vi "LinxPwmSetDutyCycle.vi"(8 "Error In":errorcluster, 9 "Duty Cycles":dbl[](array[numeric]), 10 "PWM Channels":u8[](array[numeric]), 11 "LINX Resource":T1) -> (0 "Error Out":errorcluster, 3 "LINX Resource":T1)   [LabVIEW 2014, in "LMH-LINX.lvlib" / "Local IO.lvlib"]
uses:
  Local IO.lvlib
  Type Defs/LINX Ref.ctl
  Type Defs/Platform.ctl
  Type Defs/Interface.ctl
  Device/Type Defs/LINX Device Config.ctl
  Device/Type Defs/TCP Config.ctl
  Device/Type Defs/Channels.ctl
  Utilties/Generate Error.vi
  <vilib>/myRIO/Instrument Drivers/Onboard IO/PWM/PWM.lvlib
  liblinxdevice.dll
  LMH-LINX.lvlib
  Device/Device.lvlib
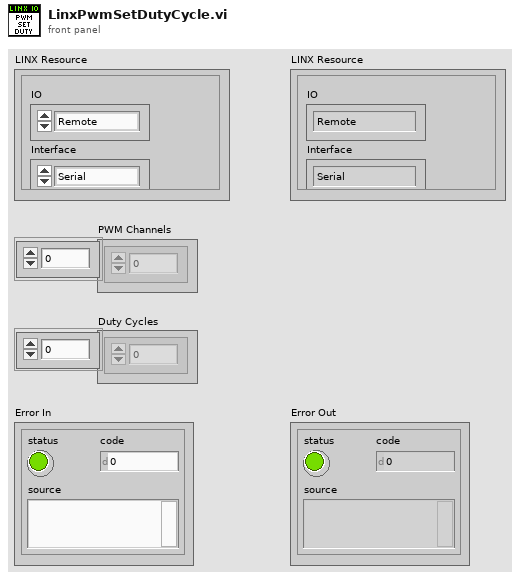
[diagram p1: front panel]
types:
  T1 = typedef "LMH-LINX.lvlib/LINX Ref.ctl" = cluster{"IO":T2, "Interface":T3, "LINX Device Config":T4}
  T2 = typedef "LMH-LINX.lvlib/Platform.ctl" = enum16{"Remote", "Local"}
  T3 = typedef "LMH-LINX.lvlib/Interface.ctl" = enum16{"Serial", "TCP"}
  T4 = typedef "LMH-LINX.lvlib/Device.lvlib/LINX Device Config.ctl" = cluster{"Interface":T3, "COM Port":refnum<visa-resource-name>, "TCP Configuration":T5, "Device Family":u8, "Device ID":u8, "Device Name":string, "TCP Ref":refnum<k5>, "Channels":T6}
  T5 = typedef "LMH-LINX.lvlib/Device.lvlib/TCP Config.ctl" = cluster{"IP Address":string, "Port":u16}
  T6 = typedef "LMH-LINX.lvlib/Channels.ctl" = cluster{"DI":u8[], "DO":u8[], "AI":u8[], "AO":u8[], "PWM":u8[], "QE":u8[], "UART":u8[], "I2C 2":u8[], "SPI":u8[], "CAN":u8[], "Servo":u8[], "AI Ref (V)":dbl, "AI Resolution (Bits)":u8, "AO Ref (V)":dbl, "AO Resolution (Bits)":u8}
  T7 = typedef "PWM.lvlib/PWM Reference.ctl" = cluster{"myRIO Reference":T8, "PWM Channels Enum":T12, "PWM Configuration":T13}
  T8 = typedef "myRIO Generic Hardware Reference.ctl" = cluster{"myRIO Model":T9, "myRIO Hardware Reference":T10}
  T9 = typedef "Hardware Version Enum.ctl" = enum16{"Unknown", "myRIO-1900", "myRIO-1950"}
  T10 = typedef "myRIO v1.0 Reference.ctl" = cluster{"Generic FPGA Reference":T11, "Allow multiple opens":bool}
  T11 = typedef "Generic FPGA Reference.ctl" = refnum<k20>
  T12 = typedef "PWM Channels Enum.ctl" = enum16{"Not Connected", "C/PWM0", "C/PWM1", "A/PWM0", "A/PWM1", "A/PWM2", "B/PWM0", "B/PWM1", "B/PWM2"}
  T13 = typedef "PWM.lvlib/PWM Configuration.ctl" = cluster{"Frequency":dbl, "Duty Cycle":dbl}
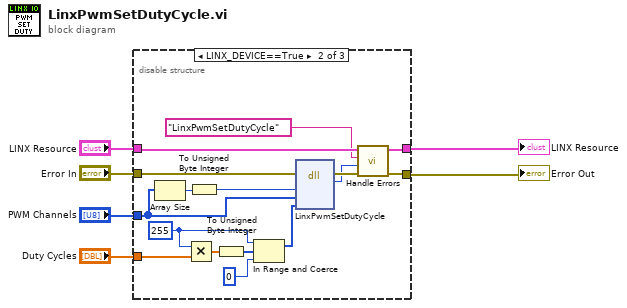
[diagram p0: block diagram]
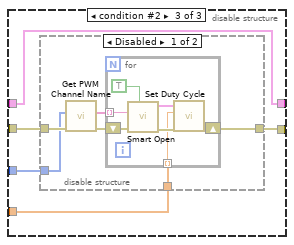
[diagram p3: hidden frame]
diagram:
  n1 = disable-structure shown="LINX_DEVICE==True" {
    disable-tunnel: "LINX Resource" -> [w8 w23 w28]
    disable-tunnel: "Error In" -> [w7 w24 w27]
    disable-tunnel: [w7 w21 w29] -> w4
    disable-tunnel: [w8 w22 w28] -> w3
    disable-tunnel: "PWM Channels" -> [_ w15 w26]
    disable-tunnel: "Duty Cycles" -> [_ w10 w25]
    frame condition #0 {
    }
    frame condition #1 (active) {
      w14 = u8 255
      n2 = Array Size(array=w15) -> (size(s)=w16:i32)
      n3 = Multiply(x=w14, y=w10) -> (x*y=w13:dbl[])
      n4 = To Unsigned Byte Integer(number=w16) -> (unsigned 8bit integer=w17:u8)
      n5 = To Unsigned Byte Integer(number=w13) -> (unsigned 8bit integer=w12:u8[])
      n6 = In Range and Coerce(upper limit=w14, x=w12, lower limit=u8 0) -> (coerced(x)=w9:u8[])  [unwired: 1 out]
      n7 = dll-call lib="liblinxdevice.*" fn="LinxPwmSetDutyCycle"(error in=w24, "numChans"=w17, "channels"=w15, "values"=w9) -> (error out=w20:errorcluster, "LinxStatus"=w19:i32)  [unwired: 5 in, 1 out]
      n8 = call "Handle Errors.vi"("Error In"=w20, "LinxStatus"=w19, "Function Name"="LinxPwmSetDutyCycle", "LINX Resource"=w23) -> ("Error Out"=w21:errorcluster, "LINX Resource"=w22:T1)  [unwired: 6 in]
    }
    frame condition #2 {
      n9 = disable-structure shown="Disabled" {
        disable-tunnel: w27 -> [w33 w43]
        disable-tunnel: [w31 w43] -> w29
        disable-tunnel: w26 -> [w32 _]
        disable-tunnel: w25 -> [w30 _]
        frame Disabled {
          n10 = call <vilib>:"Get PWM Channel Name.vi"("Error In"=w33, "PWM Channel Nums"=w32) -> ("Error Out"=w34:errorcluster, "PWM Channels"=w35:string[])  [unwired: 8 in]
          n11 = for {
            shift-right: [w42] -> w31
            shift-left: w34 -> [w41]
            tunnel: w35 -> [w40] mode=indexing
            tunnel: w30 -> [w36] mode=indexing
            n12 = call <vilib>:"Smart Open.vi"("Allow multiple opens?"=TRUE, "error in (no error)"=w41, "Channel Name"=w40) -> ("error out"=w39:errorcluster, "PWM Ref Out"=w38:T7)  [unwired: 7 in]
            n13 = call <vilib>:"Set Duty Cycle.vi"("error in (no error)"=w39, "Duty Cycle"=w36, "PWM Ref In"=w38) -> ("error out"=w42:errorcluster)  [unwired: 6 in, 1 out]
          }
        }
        frame Enabled {
          # "myRIO Support Disabled"
        }
      }
    }
  }
  "Error Out" <- w4
  "LINX Resource" <- w3
